vi "7-t-invdist.vi"(8 "error in":errorcluster caption="err in", 9 "R(t)":dbl, 10 "F(t)":dbl, 11 "p_LW":T1) -> (0 "error out":errorcluster caption="err out", 2 "t":dbl, 3 "p_LW":T1)   [LabVIEW 2010, in "lv_02.lvlib"]
uses:
  p_5E7_LW.ctl
  lv_02.lvlib
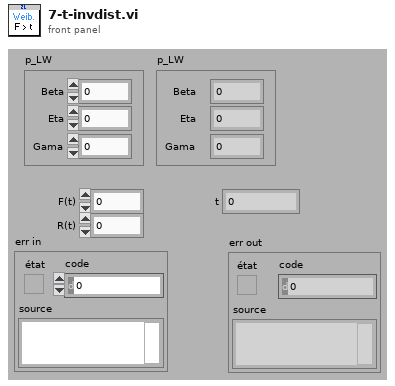
[diagram p1: front panel]
types:
  T1 = typedef "lv_02.lvlib/p_5E7_LW.ctl" = cluster{"Beta":dbl, "Eta":dbl, "Gama":dbl}
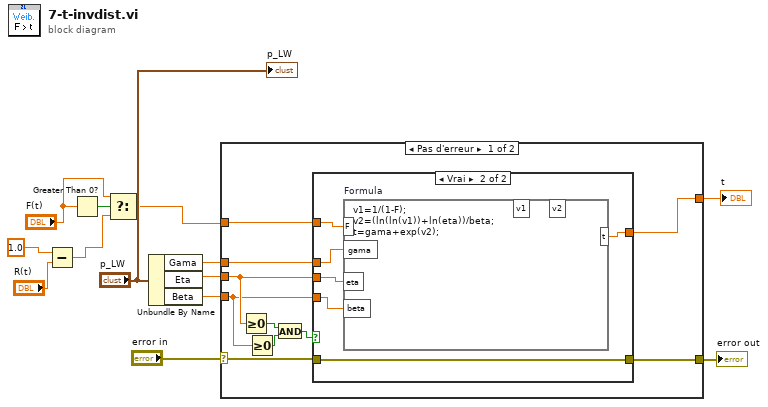
[diagram p0: block diagram]
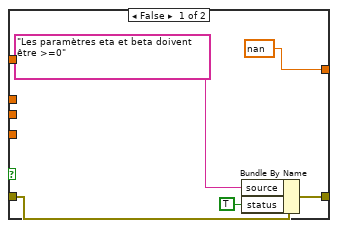
[diagram p2: hidden frame]
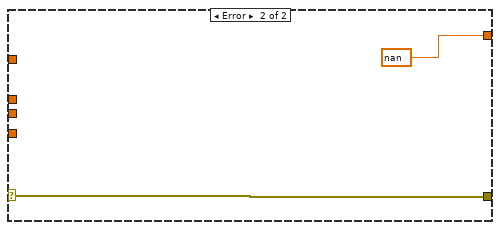
[diagram p3: hidden frame]
diagram:
  n1 = Subtract(x=1.0, y="R(t)") -> (x-y=w2:dbl)
  n2 = Greater Than 0?(x="F(t)") -> (x > 0?=w6:bool)
  n3 = Select(t="F(t)", s=w6, f=w2) -> (s? t:f=w1:dbl)
  n4 = Unbundle By Name("p_LW") -> ("Gama"=w12:dbl, "Eta"=w9:dbl, "Beta"=w10:dbl)
  n5 = case shown="Pas d'erreur" "error in" {
    selector: "error in" -> [w21 w36]
    tunnel: w1 -> [w23 _]
    tunnel: w12 -> [w22 _]
    tunnel: w10 -> [w18 _]
    tunnel: w9 -> [w19 _]
    tunnel: [w20 w36] -> w8
    tunnel: [w14 nan] -> w7
    frame No Error {
      n6 = Greater Or Equal To 0?(x=w19) -> (x >= 0?=w17:bool)
      n7 = Greater Or Equal To 0?(x=w18) -> (x >= 0?=w16:bool)
      n8 = And(x=w17, y=w16) -> (x .and. y?=w15:bool)
      n9 = case shown="Vrai" w15 {
        tunnel: w23 -> [_ w33]
        tunnel: w22 -> [_ w32]
        tunnel: w18 -> [_ w30]
        tunnel: w19 -> [_ w31]
        tunnel: w21 -> [w28 w34]
        tunnel: [w25 w34] -> w20
        tunnel: [nan w29] -> w14
        frame False {
          n10 = Bundle By Name(cluster=w28, "source"="Les paramètres eta et beta doivent  être >=0", "status"=TRUE) -> (w25:errorcluster)
        }
        frame True {
          n11 = formula code="v1=1/(1-F);\nv2=(ln(ln(v1))+ln(eta))/beta;\nt=gama+exp(v2);"("F"=w33, "gama"=w32, "eta"=w31, "beta"=w30) -> ("t"=w29:dbl)  [unwired: 2 out]
        }
      }
    }
    frame Error {
    }
  }
  "error out" <- w8
  "t" <- w7
  "p_LW" <- "p_LW"
